vi "Read Duration.vi"(11 "RetentionPolicy in":refnum<class "RetentionPolicy.lvclass">) -> (2 "Duration":i32 format="%<%H:%M:%S>t", 3 "RetentionPolicy out":refnum<class "RetentionPolicy.lvclass">)   [LabVIEW 2018, in "InfluxDB Client.lvlib" / "RetentionPolicy.lvclass"]
uses:
  RetentionPolicy.lvclass
  RetentionPolicy.lvclass/RetentionPolicy.ctl
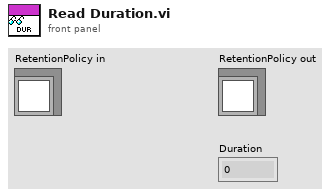
[diagram p1: front panel]
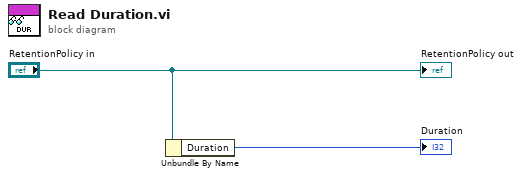
[diagram p0: block diagram]
diagram:
  n1 = Unbundle By Name("RetentionPolicy in") -> ("Duration"=→"Duration":i32)
  "RetentionPolicy out" <- "RetentionPolicy in"
